vi "fgv_tim571_setting.vi"(7 "cmd":enum16{"write", "read"}(ring), 11 "tim571_setting-data_in":T1={"TIM571 IP"="192.168.0.2", "h range"={0, 9}} {"h range" scale=-180.0..180.0}) -> (3 "tim571_setting-data_out":T1={"TIM571 IP"="192.168.0.2", "h range"={0, 9}} {"h range" scale=-180.0..180.0})   [LabVIEW 2019]
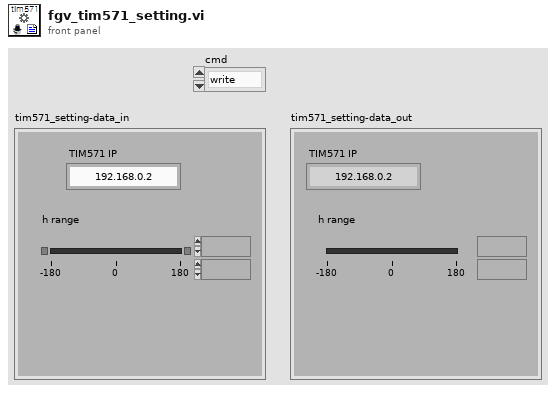
[diagram p1: front panel]
types:
  T1 = cluster{"TIM571 IP":string, "h range":cluster{i16, i16}}
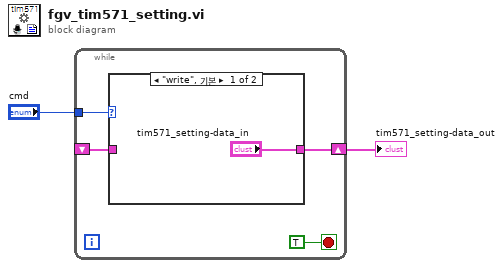
[diagram p0: block diagram]
diagram:
  n1 = while {
    tunnel: "cmd" -> [w5]
    shift-right: [w4] -> w1
    shift-left: _ -> [w3]
    stop <- TRUE stop-if-true
    n2 = case shown="\"write\", 기본" w5 {
      tunnel: ["tim571_setting-data_in" w8] -> w4
      tunnel: w3 -> [_ w8]
      frame "write", Default {
      }
      frame "read" {
      }
    }
  }
  "tim571_setting-data_out" <- w1
